vi "Delete Admin Passwordv2.vi"(8 "error in (no error)":errorcluster, 10 "index":i32, 11 "Masterv2 in":refnum<class "Masterv2.lvclass">) -> (0 "error out":errorcluster, 3 "Masterv2 out":refnum<class "Masterv2.lvclass">)   [LabVIEW 2014, in "Main Libraryv2.lvlib" / "Masterv2.lvclass"]
uses:
  Master/Masterv2.lvclass
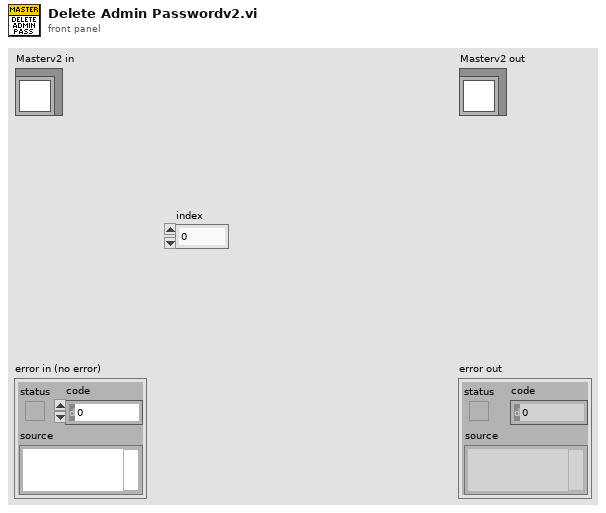
[diagram p1: front panel]
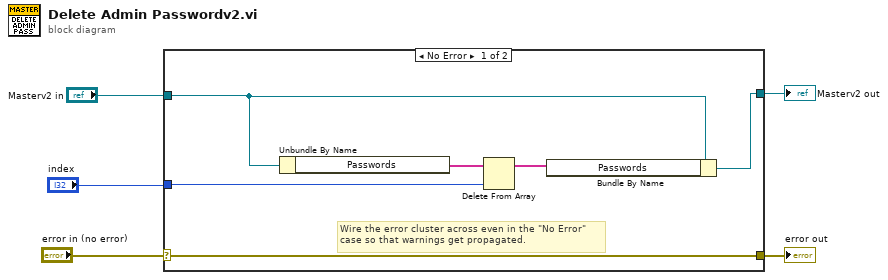
[diagram p0: block diagram]
diagram:
  n1 = case shown="No Error" "error in (no error)" {
    selector: "error in (no error)" -> [w11 w13]
    tunnel: [w11 w13] -> w4
    tunnel: [w7 w12] -> w2
    tunnel: "Masterv2 in" -> [w8 w12]
    tunnel: "index" -> [w6 _]
    frame No Error {
      # "Wire the error cluster across even in the \"No Error\"\ncase so that warnings get propagated."
      n2 = Unbundle By Name(w8) -> ("Passwords"=w10:string[])
      n3 = Delete From Array(array=w10, index=w6) -> (array with subset deleted=w9:string[])  [unwired: 1 in, 1 out]
      n4 = Bundle By Name(cluster=w8, "Passwords"=w9) -> (w7:refnum<class "Masterv2.lvclass">)
    }
    frame Error {
    }
  }
  "error out" <- w4
  "Masterv2 out" <- w2
